vi "gotowoscDoPomiaru.vi"(3 "Akcja":T2, 4 "Wybór komory":T1, 5 "Gotowoœæ":T3) -> (2 "Gotowoœæ wyjœcie":T3)   [LabVIEW 2014]
uses:
  gotowoscDoPomiaruVIs/Gotowosc.ctl
  AkcjaGFV.ctl
  parametryKomorVIs/WyborKomory.ctl
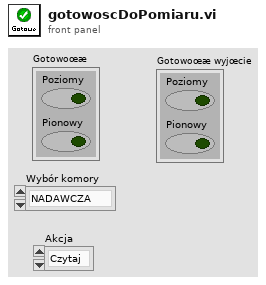
[diagram p1: front panel]
types:
  T1 = typedef "WyborKomory.ctl" = enum16{"NADAWCZA", "ODBIORCZA"}
  T2 = typedef "AkcjaGFV.ctl" = enum16{"Czytaj", "Zapisz", "Reset"}
  T3 = typedef "Gotowosc.ctl" = cluster{"Poziomy":bool, "Pionowy":bool}
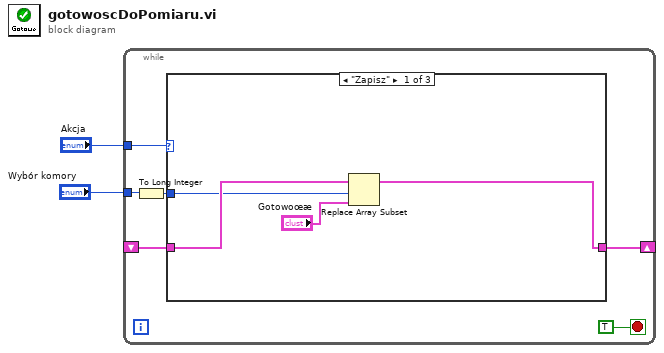
[diagram p0: block diagram]
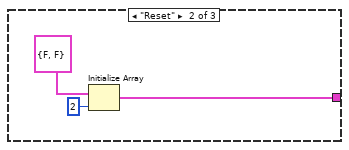
[diagram p2: hidden frame]
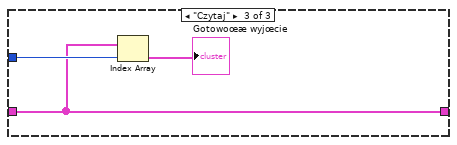
[diagram p3: hidden frame]
diagram:
  n1 = while {
    tunnel: "Akcja" -> [w7]
    shift-right: [w5] -> _
    shift-left: _ -> [w6]
    tunnel: "Wybór komory" -> [w4]
    stop <- TRUE stop-if-true
    n2 = To Long Integer(number=w4) -> (32bit integer=w3:i32)
    n3 = case shown="\"Zapisz\"" w7 {
      tunnel: w6 -> [w12 _ w16]
      tunnel: [w9 w15 w16] -> w5
      tunnel: w3 -> [w11 _ w18]
      frame "Zapisz" {
        n4 = Replace Array Subset(array=w12, new element="Gotowoœæ", index=w11) -> (w9:T3[])
      }
      frame "Reset" {
        n5 = Initialize Array(T3 {"Poziomy"=FALSE, "Pionowy"=FALSE} ("Cluster"), 2 ("dimension size")) -> (w15:T3[])
      }
      frame "Czytaj" {
        n6 = Index Array(array=w16, index=w18) -> (element=→"Gotowoœæ wyjœcie":T3)
      }
    }
  }
